vi "FPGA Resampling (50 Hz).vi"(0 "signal in":fxp<+/-,24,1>, 1 "number of channels":T3=7 items=["1"=1, "2"=2, "3"=3, "4"=4, "5"=5, "6"=6, "7"=7, "8"=8, "9"=9, "10"=10, "11"=11, "12"=12, "13"=13, "14"=14, "15"=15, "16"=16, "17"=17, "18"=18, "19"=19, "20"=20, "21"=21, "22"=22, "23"=23, "24"=24, "25"=25, "26"=26, "27"=27, "28"=28, "29"=29, "30"=30, "31"=31, "32"=32], 5 "timestamp [s]":fxp<+,64,32> format="%.42g", 7 "reference channel index (0)":u8, 9 "input valid? (T)":bool=TRUE, 12 "ready for output? (T)":bool=TRUE, 13 "samples per cycle (192)":u16=192) -> (4 "resampled data":T2, 6 "resampling info":T1={"nominal frequency"=enum."50 Hz", "resampling valid?"=FALSE, "samples per cycle"=192}, 10 "output valid?":bool, 15 "error":i32)   [LabVIEW 2014, in "NI_EP_Resample_FPGA.lvlib"]
doc: "Resamples even-time-spaced voltage and current signals into even-angle-spaced signals. The input signals must have a sample rate of 50 kHz. The output signals are synchronous with the line frequency with a constant number of samples per cycle. Use the Resampling for Power Quality VI if you want to perform resampling on the host computer. You must manually select the polymorphic instance to use.\n\nThis VI supports measuring single-bus single-line and single-bus multiple-line systems."
uses:
  <vilib>/addons/Electrical Power/PQ/Resampling/NI_EP_Resample_FPGA.lvlib
  <vilib>/addons/Electrical Power/PQ/Resampling/FPGA/subVIs/fpga_Typedef Fnom.ctl
  <vilib>/addons/Electrical Power/PQ/Resampling/FPGA/subVIs/fpga_Resampling Info.ctl
  <vilib>/addons/Electrical Power/PQ/Resampling/FPGA/subVIs/fpga_Resampled.ctl
  <vilib>/addons/Electrical Power/PQ/Resampling/FPGA/subVIs/fpga_NofCH (32ch).ctl
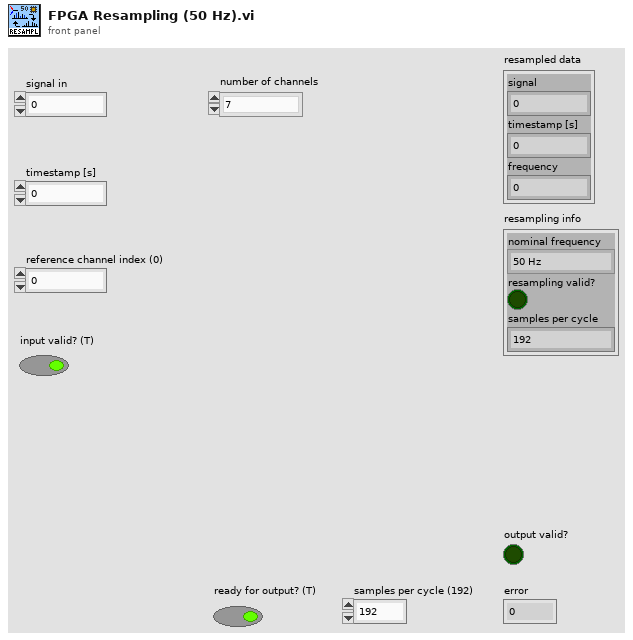
[diagram p1: front panel]
types:
  T1 = typedef "NI_EP_Resample_FPGA.lvlib/fpga_Resampling Info.ctl" = cluster{"nominal frequency":enum16{"50 Hz", "60 Hz"}, "resampling valid?":bool, "samples per cycle":u16}
  T2 = typedef "NI_EP_Resample_FPGA.lvlib/fpga_Resampled.ctl" = cluster{"signal":fxp<+/-,32,3>, "timestamp [s]":fxp<+,64,32>, "frequency":fxp<+,32,8>}
  T3 = typedef "NI_EP_Resample_FPGA.lvlib/fpga_NofCH (32ch).ctl" = u8
  T4 = typedef "NI_EP_Resample_FPGA.lvlib/fpga_Typedef Fnom.ctl" = u8
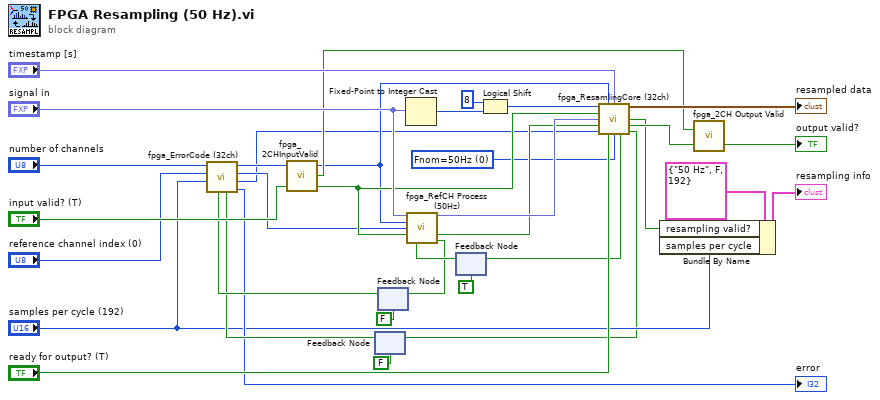
[diagram p0: block diagram]
diagram:
  w6 = T4 0 items=["Fnom=50Hz", "Fnom=60Hz"] ("Fnom")
  n1 = feedback #1(FALSE ("Ready for reference input")) -> (w9:bool)
  n2 = feedback #2(FALSE ("Ready for reference input")) -> (w11:bool)
  n3 = call <vilib>:"fpga_ErrorCode (32ch).vi"("resampling FIFO time in"=w9, "Ref filter FIFO time in"=w11, "samples per cycle"="samples per cycle (192)", "reference channel index"="reference channel index (0)", "number of channels"="number of channels") -> ("error"=→"error":i32, "samples per cycle out"=w7:u16, "ref channel index out"=w8:u8, "number of CH out"=w14:u8)  [unwired: 3 in]
  n4 = call <vilib>:"fpga_2CHInputValid.vi"("input data valid"="input valid? (T)", "Channel number"=w14) -> ("input valid"=w22:bool, "1CH?"=w24:bool, "Channel number"=w15:u8)  [unwired: 1 in]
  n5 = Fixed-Point to Integer Cast(1:"signal in") -> (0:w17:i32)
  n6 = feedback #3(TRUE ("Ready for reference input")) -> (w21:bool)
  n7 = call <vilib>:"fpga_RefCH Process (50Hz).vi"("data in <?24.1>"="signal in", "Channel number"=w15, "Reference index"=w8, "input data valid"=w22, "ready for output"=w21) -> ("Filtered Ref data"=w20:fxp<+/-,24,3>, "output valid"=w19:bool, "Timed Out"=w12:bool)  [unwired: 8 in]
  n8 = feedback-in #2(w12) -> ()
  n9 = Logical Shift(y=i8 8, x=w17) -> (x << y=w16:i32)
  n10 = call <vilib>:"fpga_ResamlingCore (32ch).vi"("data in"=w16, "Channel number"=w15, "timestamp"="timestamp [s]", "input data valid"=w22, "reference in"=w20, "input reference valid"=w19, "interpolation factor"=w7, "Ready for output"="ready for output? (T)", "Fnom"=w6) -> ("Resample data and time"=→"resampled data":T2, "resampling valid"=w4:bool, "output valid"=w23:bool, "Ready for reference input"=w26:bool, "FIFO timeout?"=w1:bool)  [unwired: 2 in]
  n11 = feedback-in #1(w1) -> ()
  n12 = feedback-in #3(w26) -> ()
  n13 = Bundle By Name(cluster=T1 {"nominal frequency"=enum."50 Hz", "resampling valid?"=FALSE, "samples per cycle"=192} ("resampling info"), "resampling valid?"=w4, "samples per cycle"="samples per cycle (192)") -> (→"resampling info":T1)
  n14 = call <vilib>:"fpga_2CH Output Valid.vi"("output valid"=w23, "1CH?"=w24) -> ("output valid"=→"output valid?":bool)  [unwired: 1 in]
